vi "DrawHover.vi"(1 "col":i32, 2 "player":i32, 3 "Board":i32[][](array[numeric])) -> (0 "2D Picture":picture)   [LabVIEW 2025]
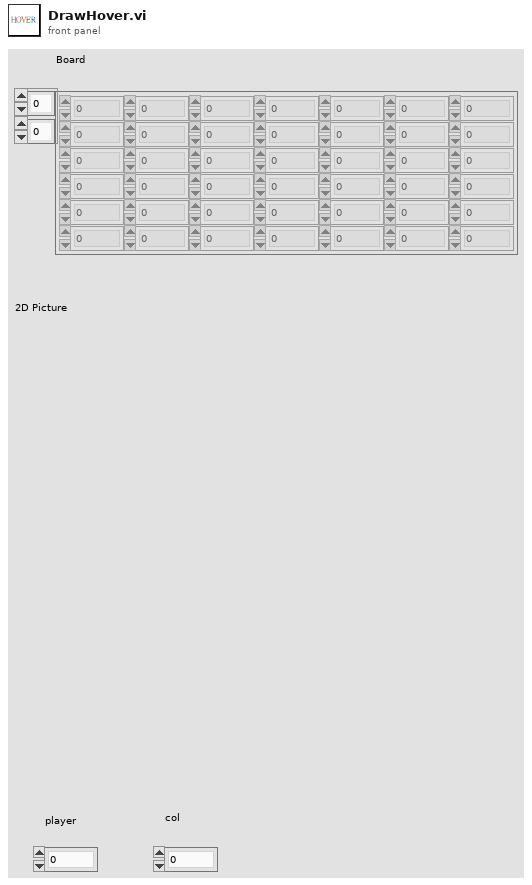
[diagram p1: front panel]
types:
  T1 = cluster{"Width":u16, "Style":enum32{"Solid", "Dash", "Dot", "DashDot", "DashDotDot"}}
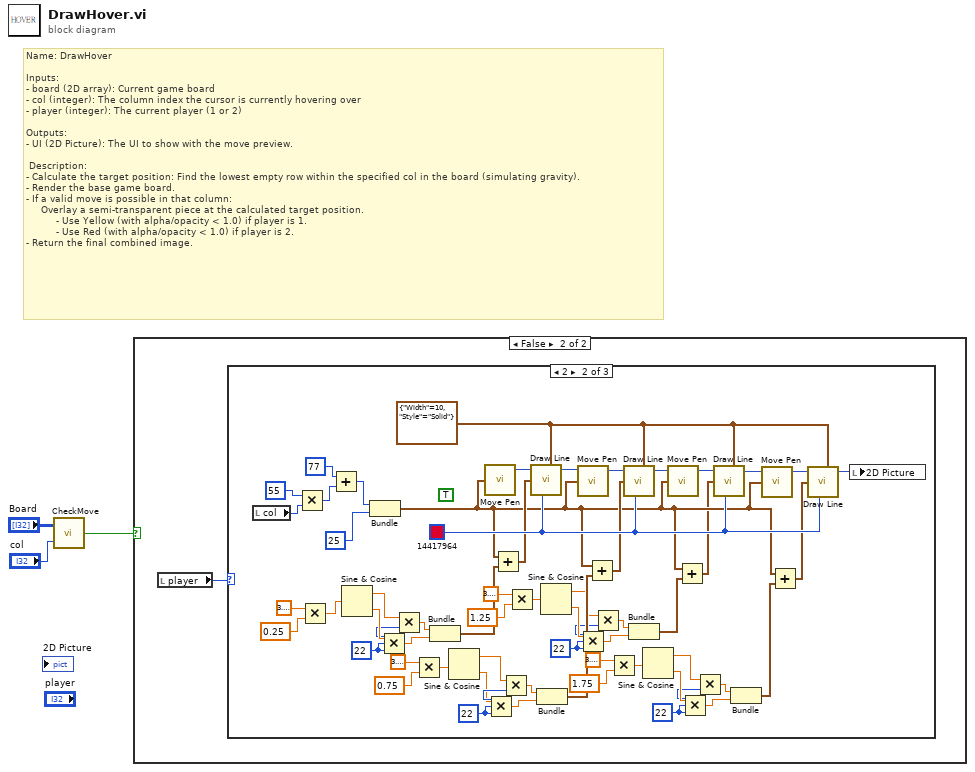
[diagram p0: block diagram]
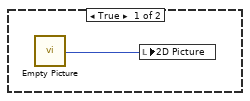
[diagram p2: hidden frame]
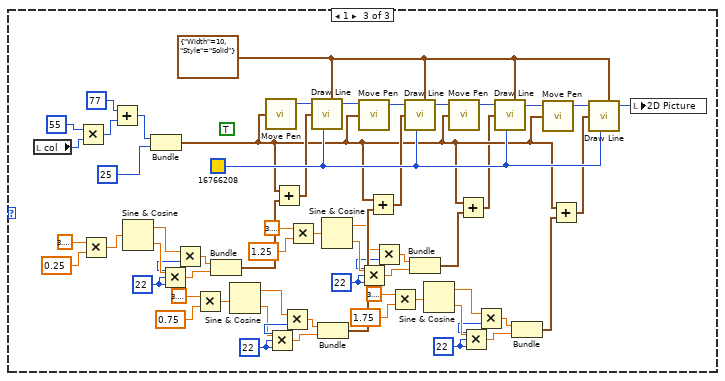
[diagram p4: hidden frame]
diagram:
  # "Name: DrawHover\n\nInputs:\n- board (2D array): Current game board\n- col (integer): The column index the cursor is currently hovering over\n- player (integer): The current player (1 or 2)\n\nOutputs:\n- UI (2D Picture): The UI to show with the move preview.\n\n Description:\n- Calculate the target position: Find the lowest empty row within the specified col in the board (simulating gravity).\n- Render the base game board.\n- If a valid move is possible in that column:\n     Overlay a semi-transparent piece at the calculated target position.\n          - Use Yellow (with alpha/opacity < 1.0) if player is 1.\n          - Use Red (with alpha/opacity < 1.0) if player is 2.\n- Return the final combined image."
  n1 = call "CheckMove.vi"("col"="col", "Board"="Board") -> ("Valid"=w1:bool)
  n2 = case shown="False" w1 {
    frame True {
      n3 = call "Empty Picture"() -> ("empty picture"=w4:picture)
      n4 = local write "2D Picture"(w4) -> ()
    }
    frame False {
      n5 = local read "player"() -> (w5:i32)
      n6 = case shown="2" w5 {
        frame 0, Default {
        }
        frame 2 {
          w8 = T1 {"Width"=10, "Style"=enum."Solid"} ("pen")
          w25 = i16 22 ("radius")
          w31 = i16 22 ("radius")
          w41 = i16 22 ("radius")
          w49 = u32 14417964 ("color(black)")
          w44 = i16 22 ("radius")
          (unwired) TRUE ("fill?(F)")
          n7 = local read "col"() -> (w58:i32)
          n8 = Multiply(x=55, y=w58) -> (x*y=w61:i32)
          n9 = Multiply(x=3.141592653589793, y=0.25) -> (x*y=w18:dbl)
          n10 = Add(x=77, y=w61) -> (x+y=w62:i32)
          n11 = Sine & Cosine(0:w18) -> (1:w45:dbl, 2:w47:dbl)
          n12 = Bundle(w62, 25) -> (w29:cluster{i32, i32})  [unwired: 1 in]
          n13 = Multiply(x=w47, y=w44) -> (x*y=w48:dbl)
          n14 = Multiply(x=w45, y=w44) -> (x*y=w46:dbl)
          n15 = Multiply(x=3.141592653589793, y=0.75) -> (x*y=w12:dbl)
          n16 = Bundle(w46, w48) -> (w43:cluster{dbl, dbl})  [unwired: 1 in]
          n17 = Sine & Cosine(0:w12) -> (1:w35:dbl, 2:w39:dbl)
          n18 = call <vilib>:"Move Pen.vi"("new position"=w29) -> ("new picture"=w57:picture)  [unwired: 4 in]
          n19 = Multiply(x=w39, y=w41) -> (x*y=w38:dbl)
          n20 = Add(x=w29, y=w43) -> (x+y=w42:cluster{dbl, dbl})
          n21 = Multiply(x=w35, y=w41) -> (x*y=w40:dbl)
          n22 = Multiply(x=3.141592653589793, y=1.25) -> (x*y=w15:dbl)
          n23 = call <vilib>:"Draw Line.vi"("picture"=w57, "end point"=w42, "color(black)"=w49, "pen"=w8) -> ("new picture"=w56:picture)  [unwired: 5 in]
          n24 = Bundle(w40, w38) -> (w36:cluster{dbl, dbl})  [unwired: 1 in]
          n25 = Sine & Cosine(0:w15) -> (1:w21:dbl, 2:w33:dbl)
          n26 = call <vilib>:"Move Pen.vi"("new position"=w29, "picture"=w56) -> ("new picture"=w55:picture)  [unwired: 3 in]
          n27 = Multiply(x=w33, y=w31) -> (x*y=w34:dbl)
          n28 = Add(x=w29, y=w36) -> (x+y=w37:cluster{dbl, dbl})
          n29 = Multiply(x=w21, y=w31) -> (x*y=w32:dbl)
          n30 = Multiply(x=3.141592653589793, y=1.75) -> (x*y=w9:dbl)
          n31 = call <vilib>:"Draw Line.vi"("picture"=w55, "end point"=w37, "color(black)"=w49, "pen"=w8) -> ("new picture"=w53:picture)  [unwired: 5 in]
          n32 = Bundle(w32, w34) -> (w30:cluster{dbl, dbl})  [unwired: 1 in]
          n33 = Sine & Cosine(0:w9) -> (1:w22:dbl, 2:w27:dbl)
          n34 = call <vilib>:"Move Pen.vi"("new position"=w29, "picture"=w53) -> ("new picture"=w54:picture)  [unwired: 3 in]
          n35 = Add(x=w29, y=w30) -> (x+y=w7:cluster{dbl, dbl})
          n36 = Multiply(x=w27, y=w25) -> (x*y=w28:dbl)
          n37 = Multiply(x=w22, y=w25) -> (x*y=w26:dbl)
          n38 = call <vilib>:"Draw Line.vi"("picture"=w54, "end point"=w7, "color(black)"=w49, "pen"=w8) -> ("new picture"=w52:picture)  [unwired: 5 in]
          n39 = Bundle(w26, w28) -> (w24:cluster{dbl, dbl})  [unwired: 1 in]
          n40 = call <vilib>:"Move Pen.vi"("new position"=w29, "picture"=w52) -> ("new picture"=w51:picture)  [unwired: 3 in]
          n41 = Add(x=w29, y=w24) -> (x+y=w23:cluster{dbl, dbl})
          n42 = call <vilib>:"Draw Line.vi"("picture"=w51, "end point"=w23, "color(black)"=w49, "pen"=w8) -> ("new picture"=w50:picture)  [unwired: 5 in]
          n43 = local write "2D Picture"(w50) -> ()
        }
        frame 1 {
          w65 = T1 {"Width"=10, "Style"=enum."Solid"} ("pen")
          w82 = i16 22 ("radius")
          w88 = i16 22 ("radius")
          w98 = i16 22 ("radius")
          w106 = u32 16766208 ("color(black)")
          w101 = i16 22 ("radius")
          (unwired) TRUE ("fill?(F)")
          n44 = local read "col"() -> (w115:i32)
          n45 = Multiply(x=55, y=w115) -> (x*y=w118:i32)
          n46 = Multiply(x=3.141592653589793, y=0.25) -> (x*y=w75:dbl)
          n47 = Add(x=77, y=w118) -> (x+y=w119:i32)
          n48 = Sine & Cosine(0:w75) -> (1:w102:dbl, 2:w104:dbl)
          n49 = Bundle(w119, 25) -> (w86:cluster{i32, i32})  [unwired: 1 in]
          n50 = Multiply(x=w104, y=w101) -> (x*y=w105:dbl)
          n51 = Multiply(x=w102, y=w101) -> (x*y=w103:dbl)
          n52 = Multiply(x=3.141592653589793, y=0.75) -> (x*y=w69:dbl)
          n53 = Bundle(w103, w105) -> (w100:cluster{dbl, dbl})  [unwired: 1 in]
          n54 = Sine & Cosine(0:w69) -> (1:w92:dbl, 2:w96:dbl)
          n55 = call <vilib>:"Move Pen.vi"("new position"=w86) -> ("new picture"=w114:picture)  [unwired: 4 in]
          n56 = Multiply(x=w96, y=w98) -> (x*y=w95:dbl)
          n57 = Add(x=w86, y=w100) -> (x+y=w99:cluster{dbl, dbl})
          n58 = Multiply(x=w92, y=w98) -> (x*y=w97:dbl)
          n59 = Multiply(x=3.141592653589793, y=1.25) -> (x*y=w72:dbl)
          n60 = call <vilib>:"Draw Line.vi"("picture"=w114, "end point"=w99, "color(black)"=w106, "pen"=w65) -> ("new picture"=w113:picture)  [unwired: 5 in]
          n61 = Bundle(w97, w95) -> (w93:cluster{dbl, dbl})  [unwired: 1 in]
          n62 = Sine & Cosine(0:w72) -> (1:w78:dbl, 2:w90:dbl)
          n63 = call <vilib>:"Move Pen.vi"("new position"=w86, "picture"=w113) -> ("new picture"=w112:picture)  [unwired: 3 in]
          n64 = Multiply(x=w90, y=w88) -> (x*y=w91:dbl)
          n65 = Add(x=w86, y=w93) -> (x+y=w94:cluster{dbl, dbl})
          n66 = Multiply(x=w78, y=w88) -> (x*y=w89:dbl)
          n67 = Multiply(x=3.141592653589793, y=1.75) -> (x*y=w66:dbl)
          n68 = call <vilib>:"Draw Line.vi"("picture"=w112, "end point"=w94, "color(black)"=w106, "pen"=w65) -> ("new picture"=w110:picture)  [unwired: 5 in]
          n69 = Bundle(w89, w91) -> (w87:cluster{dbl, dbl})  [unwired: 1 in]
          n70 = Sine & Cosine(0:w66) -> (1:w79:dbl, 2:w84:dbl)
          n71 = call <vilib>:"Move Pen.vi"("new position"=w86, "picture"=w110) -> ("new picture"=w111:picture)  [unwired: 3 in]
          n72 = Add(x=w86, y=w87) -> (x+y=w64:cluster{dbl, dbl})
          n73 = Multiply(x=w84, y=w82) -> (x*y=w85:dbl)
          n74 = Multiply(x=w79, y=w82) -> (x*y=w83:dbl)
          n75 = call <vilib>:"Draw Line.vi"("picture"=w111, "end point"=w64, "color(black)"=w106, "pen"=w65) -> ("new picture"=w109:picture)  [unwired: 5 in]
          n76 = Bundle(w83, w85) -> (w81:cluster{dbl, dbl})  [unwired: 1 in]
          n77 = call <vilib>:"Move Pen.vi"("new position"=w86, "picture"=w109) -> ("new picture"=w108:picture)  [unwired: 3 in]
          n78 = Add(x=w86, y=w81) -> (x+y=w80:cluster{dbl, dbl})
          n79 = call <vilib>:"Draw Line.vi"("picture"=w108, "end point"=w80, "color(black)"=w106, "pen"=w65) -> ("new picture"=w107:picture)  [unwired: 5 in]
          n80 = local write "2D Picture"(w107) -> ()
        }
      }
    }
  }
